vi "DestroyASCIIQueue.vi"(9 "Ready 2":bool, 10 "Ready 1":bool, 11 "Queue in":refnum<queue>) -> ()   [LabVIEW 2013]
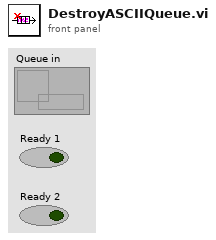
[diagram p1: front panel]
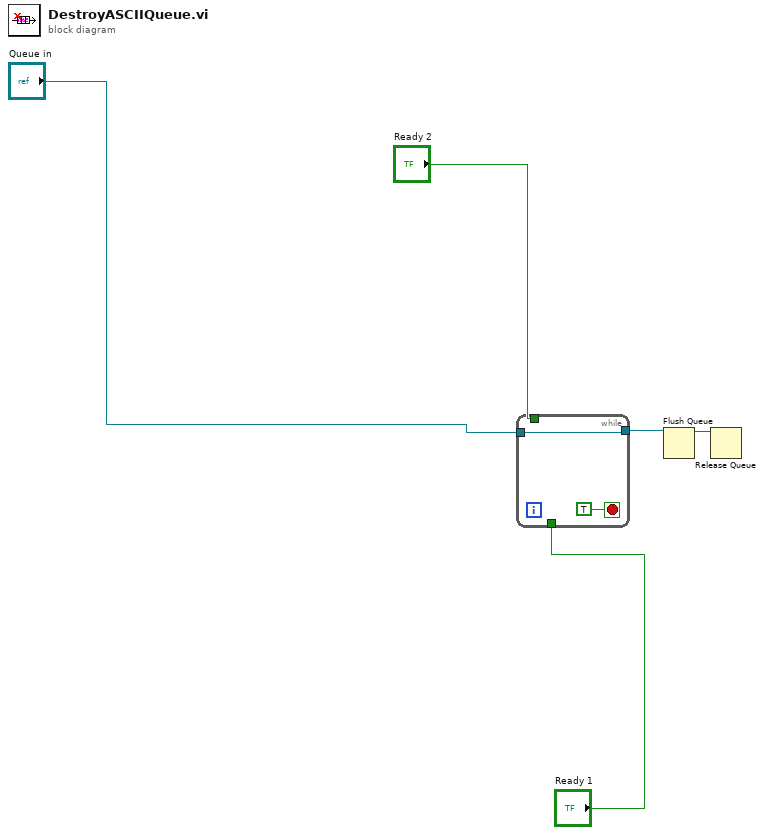
[diagram p0: block diagram]
diagram:
  n1 = while {
    tunnel: "Queue in" -> [w6]
    tunnel: [w6] -> w2
    tunnel: "Ready 2" -> [_]
    tunnel: "Ready 1" -> [_]
    stop <- TRUE stop-if-true
  }
  n2 = Flush Queue(queue=w2) -> (queue out=w1:refnum<queue>)  [unwired: 1 in, 2 out]
  n3 = Release Queue(queue=w1) -> ()  [unwired: 2 in, 3 out]
